vi "Video Stuff v08.vi"() -> ()   [LabVIEW 2009]
uses:
  <vilib>/userDefined/High Color/IMAQdx.ctl
  <vilib>/vision/NI_Vision_Development_Module.lvlib
  <vilib>/vision/driver/NI_Vision_Acquisition_Software.lvlib
panel:
  in  "Offset scale":dbl=1.51
  in  "Y":i32=1741
  in  "X":i32=777
  out "Real World Coordinates":cluster{"X":sgl, "Y":sgl} {"Y" format="%.2f"; "X" format="%.2f"}
  in  "Interpolation Type":u32(ring)=1 items=["Zero Order", "Bi-Linear", "Quadratic", "Cubic Spline"]
  in  "X Resolution":i32=640
  in  "Filter Select":T1(radio)
  in  "bin 1    bin 2":bool
  in  "Dan    Me":bool
  in  "Numeric":i32=21
  out "Occupancy Grid Square Size":dbl
  in  "LIDAR/Wheel Position Offset (in.)":dbl=60.0
  out "\"Obstickles\" y":dbl[](array[numeric])
  out "\"Obstickles\" x":dbl[](array[numeric])
  out "Small":T2(plugin-control)
  in  "Horizontal Resolution of Small Image":i32=36
  out "Super Filter":T2(plugin-control)
  in  "Color Mode":u16(ring) items=["RGB", "HSL", "HSV", "HSI"]
  in  "Blue Range":cluster{"Lower value":i32, "Upper value":i32}={"Lower value"=20, "Upper value"=255}
  in  "Green Range":cluster{"Lower value":i32, "Upper value":i32}={"Lower value"=180, "Upper value"=255}
  in  "Red Range":cluster{"Lower value":i32, "Upper value":i32}={"Lower value"=150, "Upper value"=255}
  in  "stop":bool
  out "trans":T2(plugin-control)
  out "Buffer Number":u32
  out "Live Video":T2(plugin-control)
  in  "Video Modes":i32(listbox)=20
  in  "Camera Name":T3="cam0"
  in  "Calibration File Path":path=path "C:/Documents and Settings/ekolker/My Documents/OGRE/vision/calibrationGridLargeV2.PNG"
  out "Top Image":T2(plugin-control) caption="Calibration Template"
  # "Lower:\n   YUV?\n  150, 180, 20\n   RGB?\n  240, 240, 240"
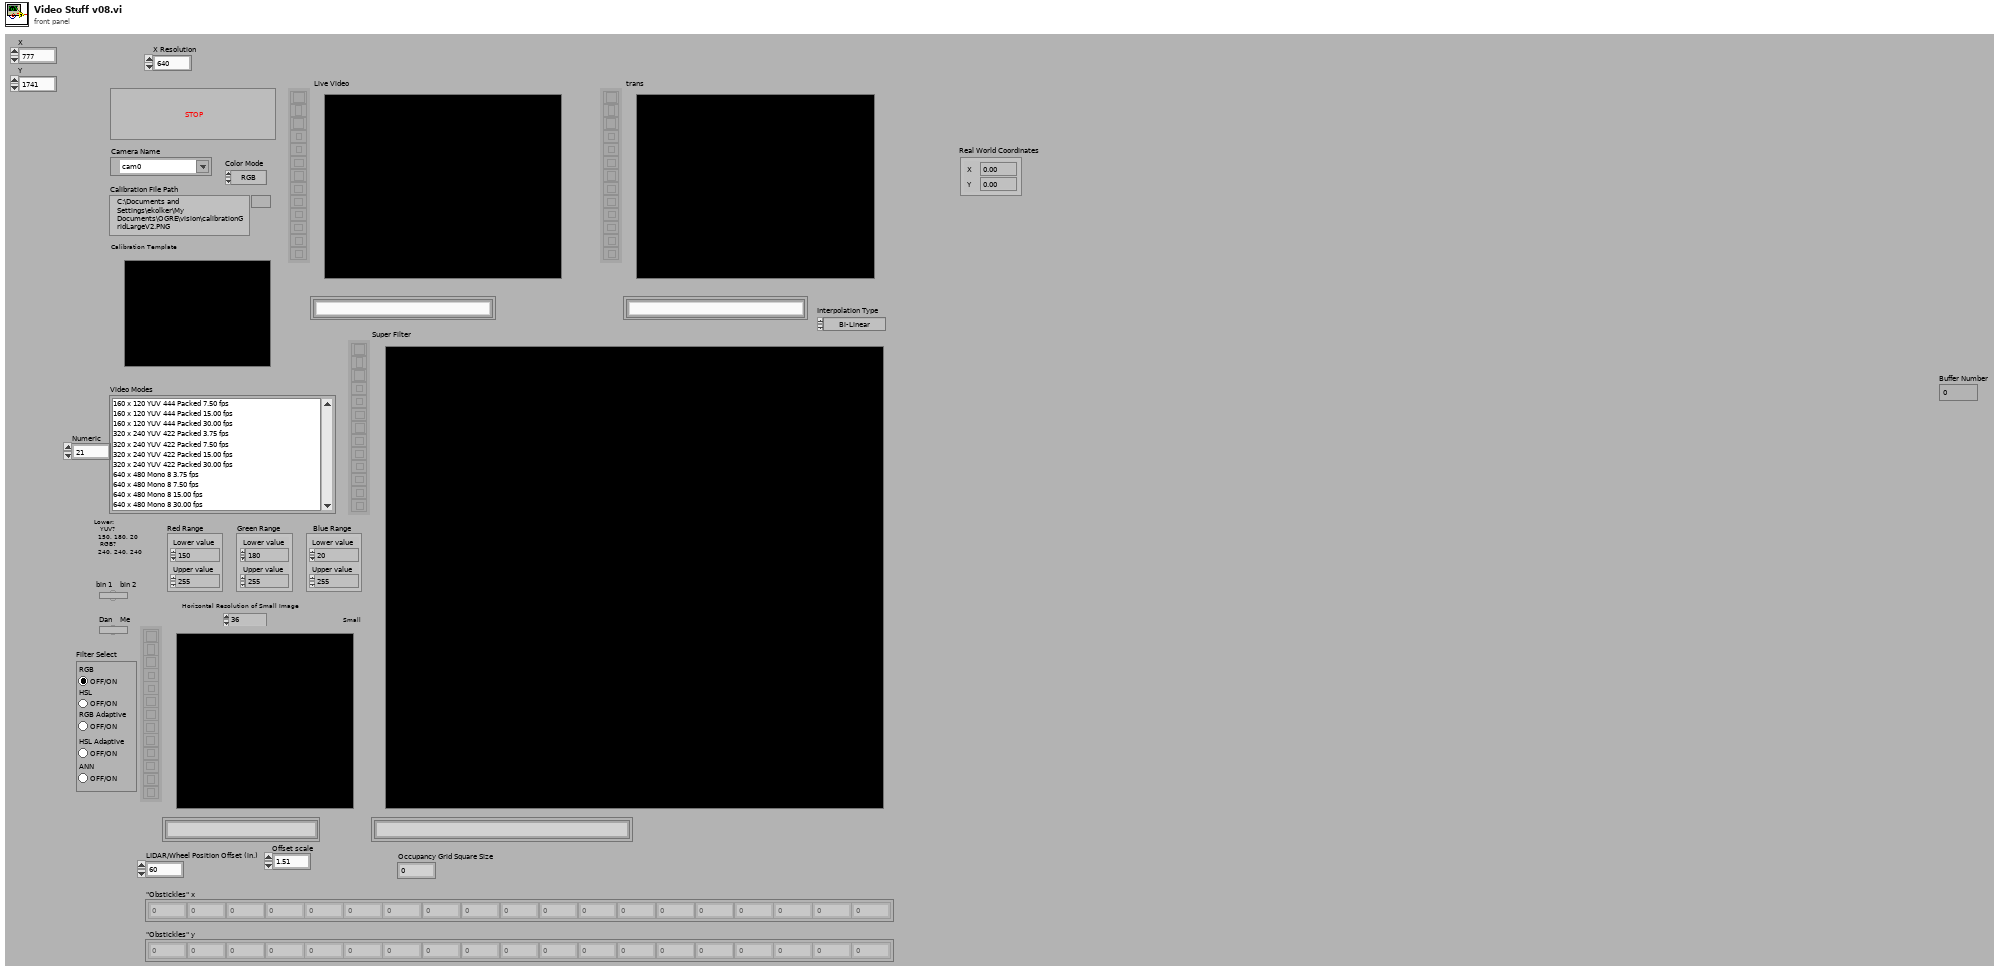
[diagram p1: front panel]
types:
  T1 = enum32{"RGB", "HSL", "RGB Adaptive", "HSL Adaptive", "ANN"}
  T2 = typedef "IMAQ Image.ctl" = refnum<image>
  T3 = typedef "IMAQdx.ctl" = refnum<k21>
  T4 = cluster{"Origin Pixel":cluster{"X":sgl, "Y":sgl}, "Angle Relative to Horizontal (deg)":sgl, "Axis Reference":u32}
  T5 = typedef "Image Type" = u32
  T6 = cluster{"X Step":sgl, "Y Step":sgl, "Unit":u32, "Threshold Range":cluster{"Lower value":sgl, "Upper value":sgl}}
  T7 = cluster{"Distortion":u32, "Corrected Image Scaling":u32, "Corrected Image Learn ROI":u32, "Learn Error Map?":bool, "Learn Correction Table?":bool}
  T8 = cluster{cluster{sgl, sgl}, "Angle Relative to Horizontal (deg)":sgl, "Axis Reference":u32}
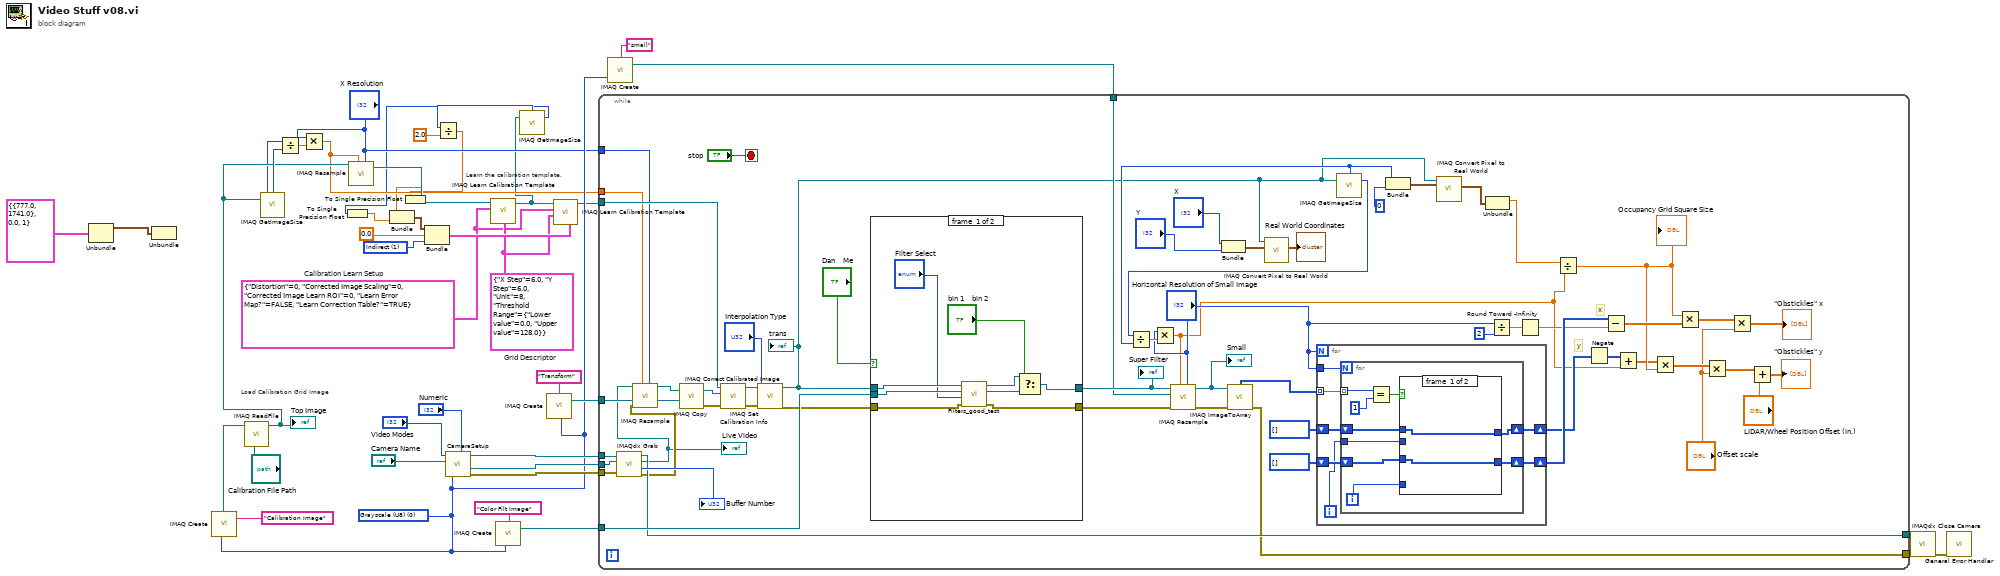
[diagram p0: block diagram]
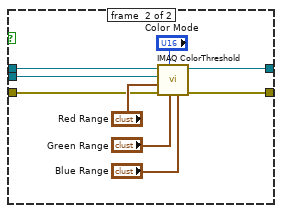
[diagram p2: hidden frame]
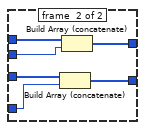
[diagram p3: hidden frame]
diagram:
  w16 = u32 1 items=["Direct", "Indirect"] ("Axis Reference")
  w29 = T5 0 items=["Grayscale (U8)", "Grayscale (I16)", "Grayscale (SGL)", "Complex (CSG)", "RGB (U32)", "HSL (U32)", "RGB (U64)", "Grayscale (U16)"] ("Image Type")
  w2 = T6 {"X Step"=6.0, "Y Step"=6.0, "Unit"=8, "Threshold Range"={"Lower value"=0.0, "Upper value"=128.0}}  # Grid Descriptor
  w1 = T7 {"Distortion"=0, "Corrected Image Scaling"=0, "Corrected Image Learn ROI"=0, "Learn Error Map?"=FALSE, "Learn Correction Table?"=TRUE}  # Calibration Learn Setup
  # "Load Calibration Grid Image"
  # "Learn the calibration template."
  n1 = Unbundle(T4 {"Origin Pixel"={"X"=777.0, "Y"=1741.0}, "Angle Relative to Horizontal (deg)"=0.0, "Axis Reference"=1} ("Calibration Axis Info")) -> ("Origin Pixel"=w7:cluster{"X":sgl, "Y":sgl})  [unwired: 2 out]
  n2 = Unbundle(w7) -> ()  [unwired: 2 out]
  n3 = call "IMAQ Create"("Image Name"="Calibration Image", "Image Type"=w29) -> ("New Image"=w32:T2)  [unwired: 2 in, 2 out]
  n4 = call "IMAQ ReadFile"("File Path"="Calibration File Path", "Image"=w32) -> ("Image Out"=w20:T2)  [unwired: 3 in, 6 out]
  "Top Image" <- w20
  n5 = call "IMAQ GetImageSize"("Image"=w20) -> ("Y Resolution"=w17:i32, "X Resolution"=w22:i32)  [unwired: 3 in, 1 out]
  n6 = Divide(x=w17, y=w22) -> (x/y=w23:dbl)
  n7 = Multiply(x="X Resolution", y=w23) -> (x*y=w18:dbl)
  n8 = call "IMAQ Resample"("X Resolution"="X Resolution", "Y Resolution"=w18, "Image Src"=w20) -> ("Image Dst Out"=w19:T2)  [unwired: 7 in, 1 out]
  n9 = call "CameraSetup.vi"("Video Modes"="Video Modes", "Camera Name"="Camera Name", "Image Type"=w29, "Numeric"="Numeric") -> ("Session Out"=w35:T3, "New Image"=w34:T2, "error out"=w33:errorcluster)  [unwired: 2 in]
  n10 = call "IMAQ Learn Calibration Template"("Grid Descriptor"=w2, "Calibration Learn Setup"=w1, "Image"=w19) -> ("Calibrated Image"=w11:T2)  [unwired: 4 in, 4 out]
  n11 = call "IMAQ Create"("Image Name"="Color Filt Image", "Image Type"=w29) -> ("New Image"=w31:T2)  [unwired: 2 in, 2 out]
  n12 = call "IMAQ GetImageSize"("Image"=w11) -> ("Y Resolution"=w6:i32, "X Resolution"=w9:i32)  [unwired: 3 in, 1 out]
  n13 = To Single Precision Float(number=w6) -> (single precision float=w5:sgl)
  n14 = Divide(x=w9, y=2.0) -> (x/y=w4:dbl)
  n15 = To Single Precision Float(number=w4) -> (single precision float=w3:sgl)
  n16 = Bundle(w3, w5) -> (w14:cluster{sgl, sgl})  [unwired: 1 in]
  n17 = Bundle(w14, "Angle Relative to Horizontal (deg)"=sgl 0.0, "Axis Reference"=w16) -> (w12:T8)  [unwired: 1 in]
  n18 = call "IMAQ Create"("Image Name"="Transform", "Image Type"=w29) -> ("New Image"=w36:T2)  [unwired: 2 in, 2 out]
  n19 = call "IMAQ Learn Calibration Template"("Calibration Axis Info"=w12, "Grid Descriptor"=w2, "Calibration Learn Setup"=w1, "Image"=w11) -> ("Calibrated Image"=w13:T2)  [unwired: 3 in, 4 out]
  n20 = call "IMAQ Create"("Image Name"="small", "Image Type"=w29) -> ("New Image"=w28:T2)  [unwired: 2 in, 2 out]
  n21 = while {
    tunnel: w13 -> [w65]
    tunnel: w36 -> [w97]
    tunnel: w35 -> [w96]
    tunnel: w34 -> [w95]
    tunnel: w33 -> [w94]
    tunnel: w31 -> [w88]
    tunnel: w28 -> [w86]
    tunnel: [w84] -> w26
    tunnel: [w83] -> w25
    tunnel: "X Resolution" -> [w49]
    tunnel: w18 -> [w50]
    stop <- "stop" stop-if-true
    # "y"
    # "x"
    n22 = call <vilib>:"IMAQdx Grab.vi"("error in"=w94, "Image In"=w95, "Session In"=w96) -> ("error out"=w68:errorcluster, "Buffer Number Out"=→"Buffer Number":u32, "Image Out"=w67:T2, "Session Out"=w84:T3)  [unwired: 1 in, 4 out]
    "Live Video" <- w67
    n23 = call "IMAQ Resample"("X Resolution"=w49, "Y Resolution"=w50, "error in (no error)"=w68, "Image Src"=w67) -> ("Image Dst Out"=w66:T2)  [unwired: 6 in, 1 out]
    n24 = call "IMAQ Copy"("Image Dst"=w97, "Image Src"=w66) -> ("error out"=w98:errorcluster, "Image Dst Out"=w101:T2)  [unwired: 4 in]
    n25 = call "IMAQ Set Calibration Info"("error in (no error)"=w98, "Image Dst"=w101, "Image Src"=w65) -> ("error out"=w99:errorcluster, "Calibrated Image"=w100:T2)  [unwired: 1 in, 6 out]
    n26 = call "IMAQ Correct Calibrated Image"("Interpolation Type"="Interpolation Type", "error in (no error)"=w99, "Image Src"=w100) -> ("error out"=w87:errorcluster, "Corrected Image"=w51:T2)  [unwired: 4 in, 3 out]
    "trans" <- w51
    n27 = case shown="False" "Dan    Me" {
      tunnel: [w110 w116] -> w93
      tunnel: [w107 w115] -> w92
      tunnel: w88 -> [w108 w114]
      tunnel: w87 -> [w111 w113]
      tunnel: w51 -> [w109 w112]
      frame #0 {
        n28 = call "Filters_good_test.vi"("error in"=w111, "Filter Select"="Filter Select", "Filter"=w108, "Input"=w109) -> ("error out"=w110:errorcluster, "Filter Binary"=w106:T2, "Filter Binary 2"=w105:T2)  [unwired: 5 in]
        n29 = Select(t=w105, s="bin 1    bin 2", f=w106) -> (s? t:f=w107:T2)
      }
      frame #1 {
        n30 = call "IMAQ ColorThreshold"("Blue or Luma or Val or Inten Range"="Blue Range", "Green or Sat Range"="Green Range", "Color Mode"="Color Mode", "error in (no error)"=w113, "Red or Hue Range"="Red Range", "Image Dst"=w114, "Image Src"=w112) -> ("error out"=w116:errorcluster, "Image Dst Out"=w115:T2)  [unwired: 3 in]
      }
    }
    "Super Filter" <- w92
    n31 = Bundle("X"="X", "Y"="Y") -> (w61:cluster{"X":i32, "Y":i32})  [unwired: 1 in]
    n32 = call "IMAQ Convert Pixel to Real World"("Pixel Coordinates"=w61, "Calibrated Image"=w51) -> ("Real World Coordinates"=→"Real World Coordinates":cluster{"X":sgl, "Y":sgl})  [unwired: 4 in, 5 out]
    n33 = call "IMAQ GetImageSize"("Image"=w51) -> ("Y Resolution"=w53:i32, "X Resolution"=w52:i32)  [unwired: 3 in, 1 out]
    n34 = Divide(x=w53, y=w52) -> (x/y=w55:dbl)
    n35 = Multiply(x="Horizontal Resolution of Small Image", y=w55) -> (x*y=w43:dbl)
    n36 = call "IMAQ Resample"("X Resolution"="Horizontal Resolution of Small Image", "Y Resolution"=w43, "error in (no error)"=w93, "Image Dst"=w86, "Image Src"=w92) -> ("error out"=w91:errorcluster, "Image Dst Out"=w90:T2)  [unwired: 5 in]
    "Small" <- w90
    n37 = call "IMAQ ImageToArray"("error in (no error)"=w91, "Image"=w90) -> ("error out"=w83:errorcluster, "Image Pixels (U8)"=w80:u8[][])  [unwired: 2 in, 3 out]
    n38 = for {
      N: "Horizontal Resolution of Small Image" -> [_]
      tunnel: "Horizontal Resolution of Small Image" -> [w127]
      tunnel: w80 -> [w126] mode=indexing
      shift-right: [w125] -> w79
      shift-left: i32[] [] -> [w124]
      shift-right: [w122] -> w72
      shift-left: i32[] [] -> [w121]
      i -> [w123]
      n39 = for {
        N: w127 -> [_]
        tunnel: w126 -> [w136] mode=indexing
        shift-right: [w132] -> w125
        shift-left: w124 -> [w131]
        tunnel: w123 -> [w130]
        shift-right: [w129] -> w122
        shift-left: w121 -> [w128]
        i -> [w134]
        n40 = Equal?(x=w136, y=u8 1) -> (x = y?=w133:bool)
        n41 = case shown="False" w133 {
          tunnel: w134 -> [_ w144]
          tunnel: [w137 w143] -> w132
          tunnel: w131 -> [w137 w142]
          tunnel: w130 -> [_ w141]
          tunnel: [w138 w140] -> w129
          tunnel: w128 -> [w138 w139]
          frame #0 {
          }
          frame #1 {
            n42 = Build Array (concatenate)(w142, w144) -> (w143:i32[])
            n43 = Build Array (concatenate)(w139, w141) -> (w140:i32[])
          }
        }
      }
    }
    n44 = Bundle("X Resolution"=w52, 0) -> (w63:cluster{"X Resolution":i32, i32})  [unwired: 1 in]
    n45 = call "IMAQ Convert Pixel to Real World"("Pixel Coordinates"=w63, "Calibrated Image"=w51) -> ("Real World Coordinates"=w57:cluster{"X":sgl, "Y":sgl})  [unwired: 4 in, 5 out]
    n46 = Unbundle(w57) -> ("X"=w56:sgl)  [unwired: 1 out]
    n47 = Divide(x="Horizontal Resolution of Small Image", y=2) -> (x/y=w71:dbl)
    n48 = Round Toward -Infinity(1:w71) -> (0:w70:dbl)
    n49 = Divide(x=w56, y=w43) -> (x/y=w77:dbl)
    "Occupancy Grid Square Size" <- w77
    n50 = Negate(x=w72) -> (-x=w73:i32[])
    n51 = Subtract(x=w79, y=w70) -> (x-y=w78:dbl[])
    n52 = Add(x=w73, y=w43) -> (x+y=w76:dbl[])
    n53 = Multiply(x=w76, y=w77) -> (x*y=w48:dbl[])
    n54 = Multiply(x=w77, y=w78) -> (x*y=w46:dbl[])
    n55 = Multiply(x=w48, y="Offset scale") -> (x*y=w47:dbl[])
    n56 = Multiply(x=w46, y="Offset scale") -> (x*y=→"\"Obstickles\" x":dbl[])
    n57 = Add(x=w47, y="LIDAR/Wheel Position Offset (in.)") -> (x+y=→"\"Obstickles\" y":dbl[])
  }
  n58 = call <vilib>:"IMAQdx Close Camera.vi"("error in"=w25, "Session In"=w26) -> ("error out"=w27:errorcluster)  [unwired: 9 out]
  n59 = call <vilib>:"General Error Handler.vi"("error in (no error)"=w27) -> ()  [unwired: 1 in, 14 out]
